vi "To String.vi"(8 "error in (no error)":errorcluster, 11 "File Path Result in":refnum<class "File Path Result.lvclass">) -> (0 "error out":errorcluster, 2 "String":string, 3 "File Path Result out":refnum<class "File Path Result.lvclass">)   [LabVIEW 2016, in "File Path Result.lvclass"]
uses:
  File Path Result.lvclass
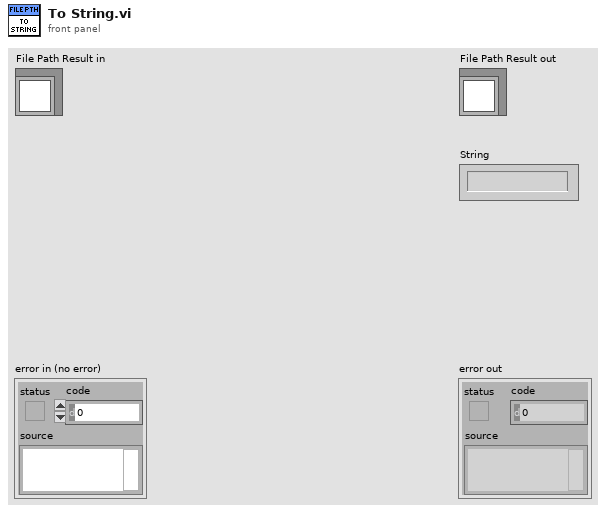
[diagram p1: front panel]
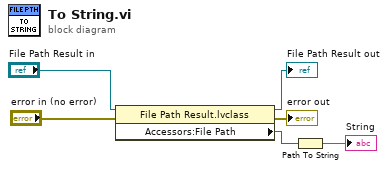
[diagram p0: block diagram]
diagram:
  n1 = property class="File Path Result.lvclass"(reference="File Path Result in", error in="error in (no error)") -> (reference out=→"File Path Result out":refnum<class "File Path Result.lvclass">, error out=→"error out":errorcluster, "Accessors:File Path"=w2:path)
  n2 = Path To String(path=w2) -> (string=→"String":string)
